vi "initialise.vi"(8 "error in (no error)":errorcluster, 11 "GenericPlugin in":refnum<class "FPGAWrapperMH120124RAPS_PXI7813R.lvclass">) -> (0 "error out":errorcluster, 3 "GenericPlugin out":refnum<class "FPGAWrapperMH120124RAPS_PXI7813R.lvclass">)   [LabVIEW 2010, in "FPGAWrapperMH120124RAPS_PXI7813R.lvclass"]
doc: "The dynamic dispatch-version of this VI initalises the plug-in object by allocating and initalising any dynamic resources need."
uses:
  FPGAWrapperMH120124RAPS_PXI7813R.lvclass
  GenericFPGAWrapper/GenericFPGAWrapper/GenericFPGAWrapper.lvclass
  grabber/command_enum.ctl
  FPGAWrapperMH120124RAPS_PXI7813R.lvclass/FPGAWrapperMH120124RAPS_PXI7813R.ctl
  class_data.vi
  common/classes/ErrorController/ErrorController/class_data.vi
  common/classes/ErrorController/ErrorController/ErrorController.lvclass
panel:
  out "appended path":path
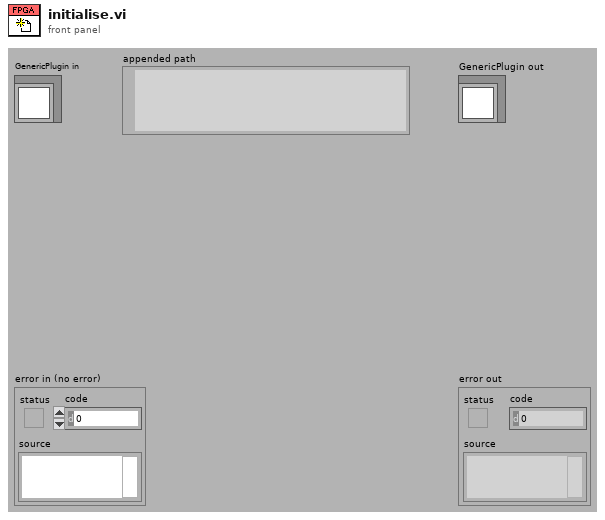
[diagram p1: front panel]
types:
  T1 = typedef "command_enum.ctl" = enum8{"NULL", "update", "start", "stop", "reset", "shut-down"}
  T2 = typedef "configuration_cluster_raps.ctl" = cluster{"DDS board initialization parameters":T3, "OSK select":bool, "AOD equilibration time":dbl, "AOD center frequ. (Hz)":dbl, "AOD Bandwidth":dbl, "inverse?":string}
  T3 = typedef "DDS_board_init_cluster.ctl" = cluster{"Bypass PLL":bool, "PLL Range":bool, "Update Clock":bool, "Triangle ":bool, "SDO Active":bool, "LSB First":bool, "OSK Int":bool, "Output Shaped Keying Enable":bool, "Bypass Sinc":bool, "Digital Part":bool, "OutPut DAC":bool, "Control DAC":bool, "Comparator":bool, "Modus":u8, "Multiplier Value":u8}
  T4 = typedef "settings_cluster_raps.ctl" = cluster{"number of pixels":i32, "iterations per pixel":i32, "iterations per subpixel":i32, "maximum bit-depth":i8, "AOD center freq. (Hz)":dbl, "AOD bandwidth freq. (Hz)":dbl, "AOD amplitude":u16, "pixel dwell time":dbl, "AOD equilibration time":dbl, "ra trajectory pixels (data/pixels transfered)":u32, "pattern type":i8, "ellipsoid parameter cluster":T5, "pixel values cluster":T6, "offset (Hz)":dbl[], "RAPS array":u64[], "DDS board initialization parameters":T3}
  T5 = typedef "ellipsoid_parameters_cluster.ctl" = cluster{"a":fxp<+/-,16,1>, "b":fxp<+/-,16,1>, "c":fxp<+/-,16,1>, "d":fxp<+/-,16,1>, "e":fxp<+/-,24,16>, "k":u16, "width":fxp<+,16,16>}
  T6 = typedef "channels_cluster.ctl" = cluster{"channel 0":u32, "channel 1":u32, "channel 2":u32, "channel 3":u32}
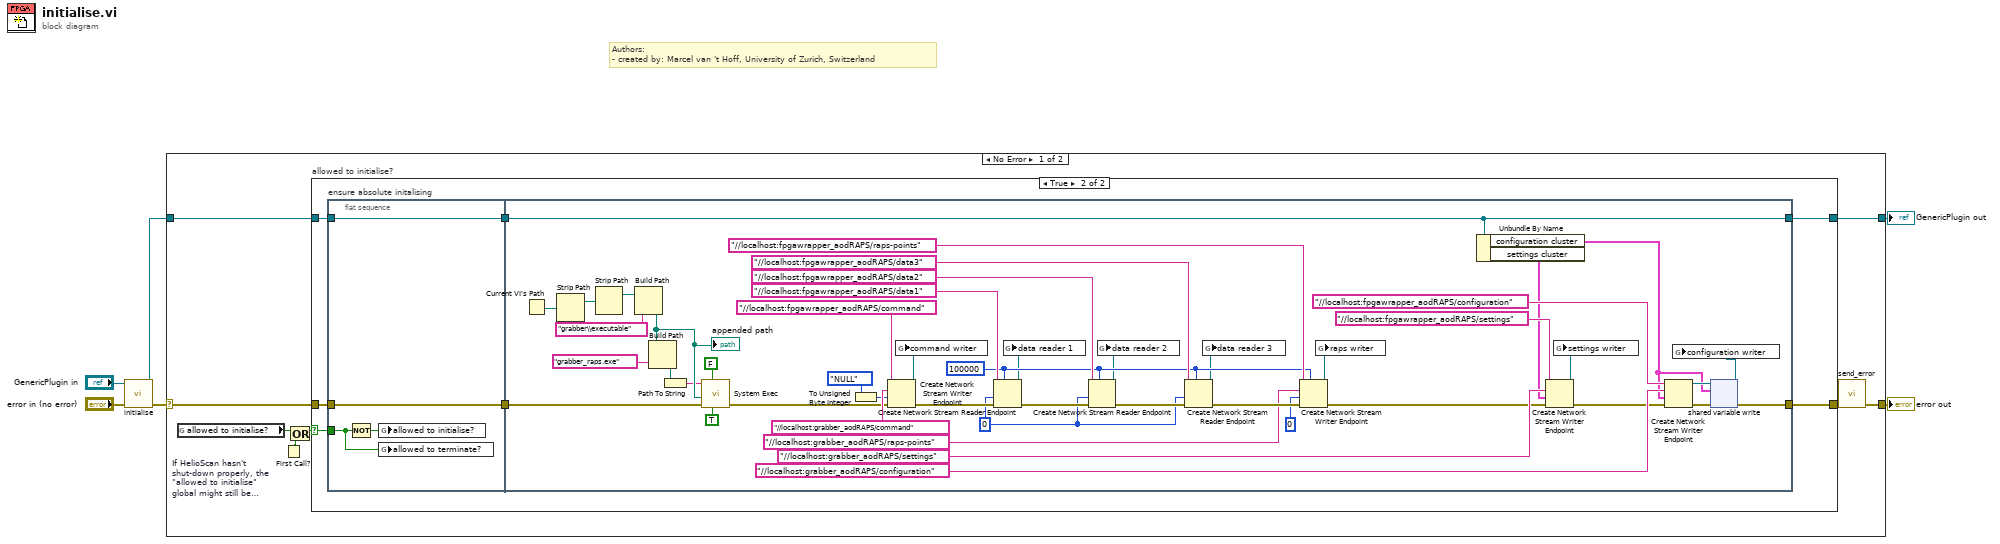
[diagram p0: block diagram]
diagram:
  # "Authors: \n- created by: Marcel van 't Hoff, University of Zurich, Switzerland"
  n1 = call-parent "initialise.vi"("error in (no error)"="error in (no error)", "GenericPlugin in"="GenericPlugin in") -> ("error out"=w4:errorcluster, "GenericPlugin out"=w3:refnum<class "FPGAWrapperMH120124RAPS_PXI7813R.lvclass">)  [unwired: 8 in]
  n2 = case shown="No Error" w4 {
    selector: w4 -> [w13 w76]
    tunnel: w3 -> [w12 w75]
    tunnel: [w14 w75] -> w1
    tunnel: [w8 w76] -> w2
    frame No Error {
      n3 = global read "class_data.vi" "allowed to initialise?"() -> (w10:bool)
      n4 = First Call? "If HelioScan hasn't shut-down properly, the \"allowed to initialise\" global might still be false..."() -> (First Call?: T/F=w11:bool)
      n5 = Or(x=w10, y=w11) -> (x .or. y?=w9:bool)
      n6 = case "allowed to initialise?" shown="True" w9 {
        selector: w9 -> [_ w20]
        tunnel: [w15 w17] -> w14
        tunnel: w12 -> [w15 w21]
        tunnel: [w16 w22] -> w7
        tunnel: w13 -> [w16 w23]
        frame False {
        }
        frame True {
          n7 = flat-sequence "ensure absolute initalising" {
            tunnel: w20 -> [w24]
            tunnel: w21 -> [w26]
            tunnel: w23 -> [w27]
            tunnel: [w27] -> w19
            tunnel: [w26] -> w18
            tunnel: [w61] -> w22
            tunnel: w19 -> [w74]
            tunnel: w18 -> [w28]
            tunnel: [w28] -> w17
            frame #0 {
              n8 = Not(x=w24) -> (.not. x?=w25:bool)
              n9 = global write "class_data.vi" "allowed to initialise?"(w25) -> ()
              n10 = global write "class_data.vi" "allowed to terminate?"(w24) -> ()
            }
            frame #1 {
              w46 = 100000 ("reader buffer size")
              w54 = u32 0
              n11 = Current VI's Path() -> (path=w34:path)
              n12 = Strip Path(path=w34) -> (stripped path=w31:path)  [unwired: 1 out]
              n13 = Strip Path(path=w31) -> (stripped path=w30:path)  [unwired: 1 out]
              n14 = Build Path(base path=w30, name or relative path="grabber\\executable") -> (appended path=w36:path)
              "appended path" <- w36
              n15 = Build Path(base path=w36, name or relative path="grabber_raps.exe" ("command line")) -> (appended path=w29:path)
              n16 = Path To String(path=w29) -> (string=w35:string)
              n17 = call <vilib>:"System Exec.vi"("run minimized? (F)"=TRUE, "wait until completion? (T)"=FALSE, "error in (no error)"=w74, "working directory"=w36, "command line"=w35) -> ("error out"=w62:errorcluster)  [unwired: 3 in, 3 out]
              n18 = To Unsigned Byte Integer(number=command_enum."NULL" ("command")) -> (unsigned 8bit integer=w52:u8)
              n19 = Create Network Stream Writer Endpoint(8:w62, 9:w52, 10:"//localhost:grabber_aodRAPS/command" ("writer name"), 11:"//localhost:fpgawrapper_aodRAPS/command" ("writer name")) -> (0:w65:errorcluster, 3:w45:refnum<k21>)  [unwired: 2 in]
              n20 = global write "class_data.vi" "command writer"(w45) -> ()
              n21 = Create Network Stream Reader Endpoint(7:w46, 8:w65, 9:w54, 11:"//localhost:fpgawrapper_aodRAPS/data1" ("reader url")) -> (0:w57:errorcluster, 3:w44:refnum<k21>)  [unwired: 2 in]
              n22 = global write "class_data.vi" "data reader 1"(w44) -> ()
              n23 = Create Network Stream Reader Endpoint(7:w46, 8:w57, 9:w54, 11:"//localhost:fpgawrapper_aodRAPS/data2" ("reader url")) -> (0:w58:errorcluster, 3:w43:refnum<k21>)  [unwired: 2 in]
              n24 = global write "class_data.vi" "data reader 2"(w43) -> ()
              n25 = Create Network Stream Reader Endpoint(7:w46, 8:w58, 9:w54, 11:"//localhost:fpgawrapper_aodRAPS/data3" ("reader url")) -> (0:w51:errorcluster, 3:w42:refnum<k21>)  [unwired: 2 in]
              n26 = global write "class_data.vi" "data reader 3"(w42) -> ()
              n27 = Create Network Stream Writer Endpoint(7:w46, 8:w51, 9:u64 0, 10:"//localhost:grabber_aodRAPS/raps-points" ("writer name"), 11:"//localhost:fpgawrapper_aodRAPS/raps-points" ("writer name")) -> (0:w50:errorcluster, 3:w41:refnum<k21>)  [unwired: 1 in]
              n28 = global write "class_data.vi" "raps writer"(w41) -> ()
              n29 = Unbundle By Name(w28) -> ("configuration cluster"=w60:T2, "settings cluster"=w59:T4)
              n30 = Create Network Stream Writer Endpoint(8:w50, 9:w59, 10:"//localhost:grabber_aodRAPS/settings" ("writer name"), 11:"//localhost:fpgawrapper_aodRAPS/settings" ("writer name")) -> (0:w69:errorcluster, 3:w39:refnum<k21>)  [unwired: 2 in]
              n31 = global write "class_data.vi" "settings writer"(w39) -> ()
              n32 = Create Network Stream Writer Endpoint(8:w69, 9:w60, 10:"//localhost:grabber_aodRAPS/configuration" ("reader url"), 11:"//localhost:fpgawrapper_aodRAPS/configuration" ("writer name")) -> (0:w68:errorcluster, 3:w67:refnum<k21>)  [unwired: 2 in]
              n33 = shared-variable-write(w67, w68, w60) -> (w40:refnum<k21>, w61:errorcluster)  [unwired: 1 in, 1 out]
              n34 = global write "class_data.vi" "configuration writer"(w40) -> ()
            }
          }
        }
      }
      n35 = call "send_error.vi"("error in (no error)"=w7) -> ("error out"=w8:errorcluster)  [unwired: 10 in]
    }
    frame Error {
    }
  }
  "error out" <- w2
  "GenericPlugin out" <- w1
